vi "IsModel8743.vi"(8 "error in":errorcluster, 11 "Model / Serial":string) -> (0 "error out":errorcluster, 3 "Boolean":bool)   [LabVIEW 2018]
uses:
  <vilib>/regexp/Match Regular Expression.xnode
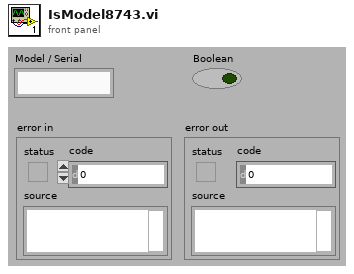
[diagram p1: front panel]
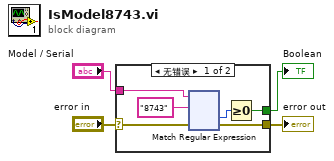
[diagram p0: block diagram]
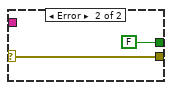
[diagram p2: hidden frame]
diagram:
  n1 = case shown="无错误" "error in" {
    selector: "error in" -> [w5 w126]
    tunnel: [w10 FALSE] -> w4
    tunnel: [w8 w126] -> w3
    tunnel: "Model / Serial" -> [w6 _]
    frame No Error {
      n2 = xnode "Match Regular Expression"("输入字符串"=w6, "正则表达式"="8743" ("regular expression"), "错误输入"=w5) -> ("匹配后偏移量"=w9:i32, "错误输出"=w8:errorcluster)  [unwired: 3 in, 3 out]
      n3 = Greater Or Equal To 0?(x=w9) -> (x >= 0?=w10:bool)
    }
    frame Error {
    }
  }
  "Boolean" <- w4
  "error out" <- w3
